vi "ZCAN_InitCAN(PCIeFD ).vi"(4 "error in (no error)":errorcluster caption="错误输入（无错误）", 5 "PCIECANFD系列初始化参数":T1, 6 "can_index":u32, 7 "device_hande":u32) -> (0 "error out":errorcluster caption="错误输出", 2 "can_index_handle":u32)   [LabVIEW 2018]
doc: "用于设置CAN通道的初始化参数。\n\n参数包括：波特率（自定义波特率）、滤波、工作模式；\n\n适用的设备：PCIE-CANFD-100U、PCIE-CANFD-200U、PCIE-CANFD-400U。"
uses:
  zlgcan_labview_20220510/zlgcan_demo_EU/bin/zlgcan_wrap.dll
  data_type/ZCAN_InitCAN_setting_PCIEFD.ctl
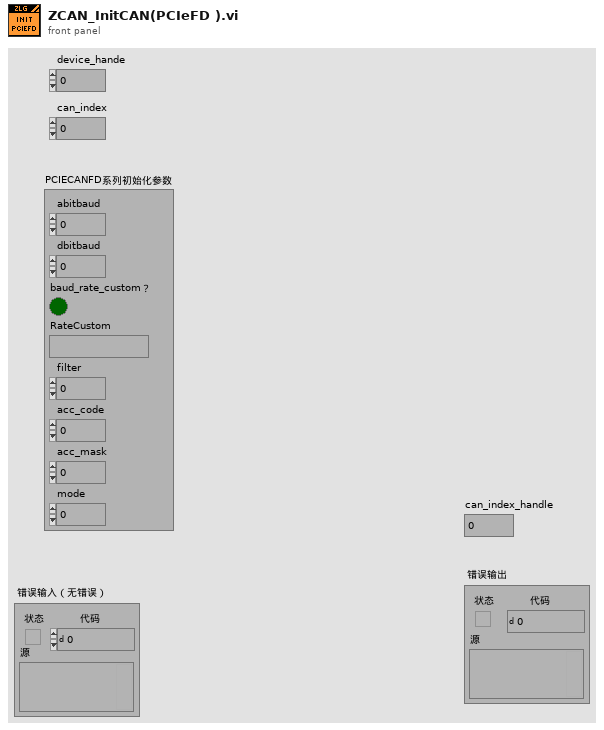
[diagram p1: front panel]
types:
  T1 = typedef "ZCAN_InitCAN_setting_PCIEFD.ctl" = cluster{"abitbaud":u32, "dbitbaud":u32, "baud_rate_custom？":bool, "RateCustom":string, "filter":u8, "acc_code":u32, "acc_mask":u32, "mode":u8}
  T2 = cluster{"can_type":u32, "acc_code":u32, "acc_mask":u32, "can_type":u32, "can_type":u32, "can_type":u32, "filter":u8, u8, "pad":u16, "reserved":u32}
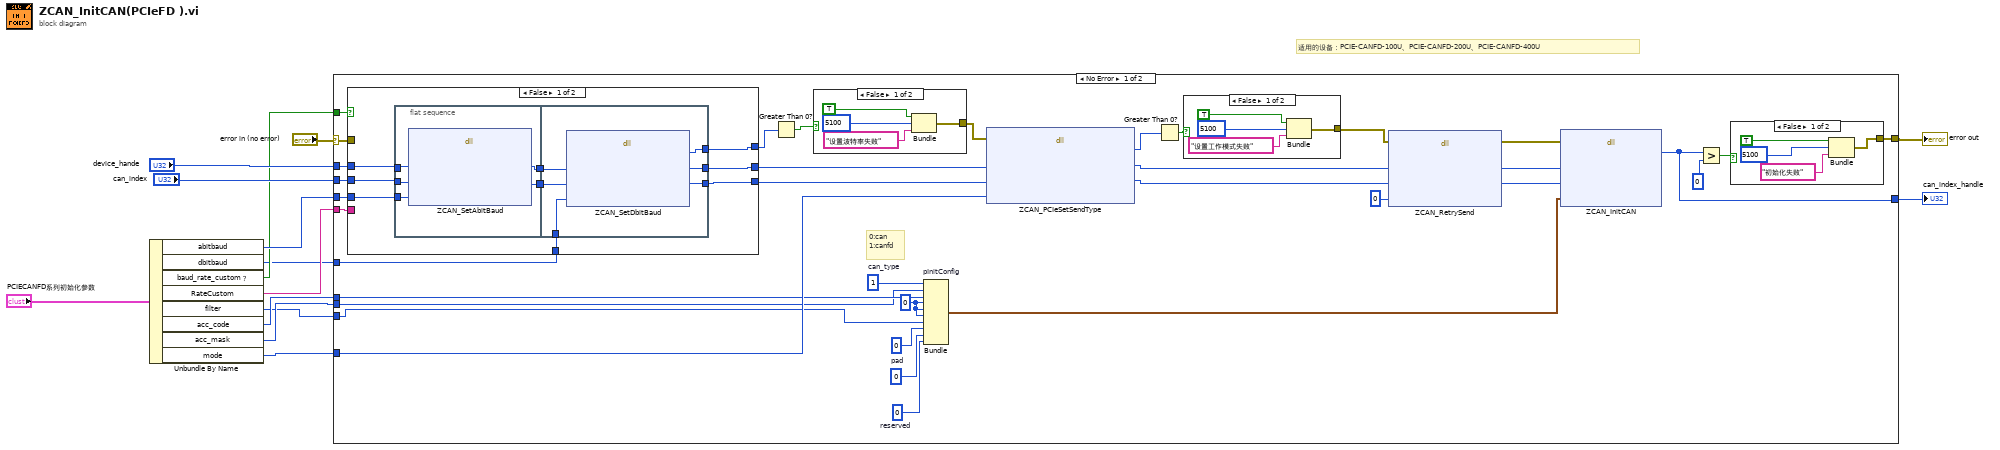
[diagram p0: block diagram]
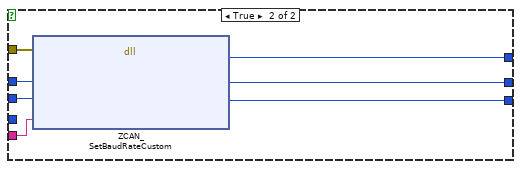
[diagram p5: hidden frame]
diagram:
  # "适用的设备：PCIE-CANFD-100U、PCIE-CANFD-200U、PCIE-CANFD-400U"
  n1 = Unbundle By Name("PCIECANFD系列初始化参数") -> ("abitbaud"=w9:u32, "dbitbaud"=w1:u32, "baud_rate_custom？"=w8:bool, "RateCustom"=w7:string, "filter"=w4:u8, "acc_code"=w6:u32, "acc_mask"=w5:u32, "mode"=w3:u8)
  n2 = case shown="No Error" "error in (no error)" {
    selector: "error in (no error)" -> [w44 w89]
    tunnel: [w40 w89] -> w13
    tunnel: w8 -> [w49 _]
    tunnel: "device_hande" -> [w48 _]
    tunnel: "can_index" -> [w47 _]
    tunnel: w9 -> [w46 _]
    tunnel: w7 -> [w45 _]
    tunnel: [w41 _] -> w12
    tunnel: w6 -> [w18 _]
    tunnel: w5 -> [w17 _]
    tunnel: w4 -> [w16 _]
    tunnel: w3 -> [w39 _]
    tunnel: w1 -> [w15 _]
    frame No Error {
      w22 = u32 0  # reserved
      w23 = u16 0  # pad
      w21 = u32 0 ("can_type")
      w24 = u32 1  # can_type
      # "0:can \n1:canfd"
      n3 = case shown="False" w49 {
        tunnel: w48 -> [w68 w88]
        tunnel: w47 -> [w67 w87]
        tunnel: w46 -> [w66 _]
        tunnel: w45 -> [_ w82]
        tunnel: [w63 w86] -> w37
        tunnel: [w62 w85] -> w38
        tunnel: w44 -> [_ w84]
        tunnel: [w64 w83] -> w36
        tunnel: w15 -> [w65 _]
        frame False {
          n4 = flat-sequence {
            tunnel: w68 -> [w73]
            tunnel: w67 -> [w72]
            tunnel: [w75] -> w70
            tunnel: [w74] -> w69
            tunnel: w66 -> [w71]
            tunnel: w70 -> [w81]
            tunnel: w69 -> [w80]
            tunnel: [w79] -> w64
            tunnel: [w78] -> w63
            tunnel: [w77] -> w62
            tunnel: w65 -> [w76]
            frame #0 {
              n5 = dll-call lib="C:/Users/admin/Desktop/zlgcan_labview_20220510/zlgcan_demo_EU/bin/zlgcan_wrap.dll" fn="ZCAN_SetAbitBaud" label="设置仲裁域波特率"("device_hande"=w73, "can_index"=w72, "abitbaud"=w71) -> ("device_hande"=w75:u32, "can_index"=w74:u32)  [unwired: 5 in, 2 out]
            }
            frame #1 {
              n6 = dll-call lib="C:/Users/admin/Desktop/zlgcan_labview_20220510/zlgcan_demo_EU/bin/zlgcan_wrap.dll" fn="ZCAN_SetDbitBaud" label="设置数据域波特率"("device_hande"=w81, "can_index"=w80, "dbitbaud"=w76) -> ("return"=w79:u32, "device_hande"=w78:u32, "can_index"=w77:u32)  [unwired: 4 in, 2 out]
            }
          }
        }
        frame True {
          n7 = dll-call lib="C:/Users/admin/Desktop/zlgcan_labview_20220510/zlgcan_demo_EU/bin/zlgcan_wrap.dll" fn="ZCAN_SetBaudRateCustom"(error in=w84, "device_handle"=w88, "can_index"=w87, "RateCustom"=w82) -> ("return"=w83:u32, "device_handle"=w86:u32, "can_index"=w85:u32)  [unwired: 3 in, 2 out]
        }
      }
      n8 = Greater Than 0?(x=w36) -> (x > 0?=w35:bool)
      n9 = case shown="False" w35 {
        tunnel: [w58 _] -> w34
        frame False {
          n10 = Bundle("status"=TRUE, "code"=5100, "消息"="设置波特率失败") -> (w58:cluster{"status":bool, "code":i32, "消息":string})  [unwired: 1 in]
        }
        frame True {
        }
      }
      n11 = Bundle "pInitConfig"("can_type"=w24, "acc_code"=w18, "acc_mask"=w17, "can_type"=w21, "can_type"=w21, "can_type"=w21, "filter"=w16, u8 0, "pad"=w23, "reserved"=w22) -> (w19:T2)  [unwired: 1 in]
      n12 = dll-call lib="C:/Users/admin/Desktop/zlgcan_labview_20220510/zlgcan_demo_EU/bin/zlgcan_wrap.dll" fn="ZCAN_PCIeSetSendType" ("ZCAN_SetBaudRateCustom")(error in=w34, "device_handle"=w37, "can_index"=w38, "mode"=w39) -> ("return"=w33:u32, "device_handle"=w28:u32, "can_index"=w27:u32)  [unwired: 3 in, 2 out]
      n13 = Greater Than 0?(x=w33) -> (x > 0?=w32:bool)
      n14 = case shown="False" w32 {
        tunnel: [w50 _] -> w31
        frame False {
          n15 = Bundle("status"=TRUE, "code"=5100, "消息"="设置工作模式失败") -> (w50:cluster{"status":bool, "code":i32, "消息":string})  [unwired: 1 in]
        }
        frame True {
        }
      }
      n16 = dll-call lib="C:/Users/admin/Desktop/zlgcan_labview_20220510/zlgcan_demo_EU/bin/zlgcan_wrap.dll" fn="ZCAN_RetrySend" ("ZCAN_SetBaudRateCustom")(error in=w31, "device_handle"=w28, "can_index"=w27, "retry_send"=u32 0) -> (error out=w29:errorcluster, "device_handle"=w26:u32, "can_index"=w25:u32)  [unwired: 4 in, 1 out]
      n17 = dll-call lib="C:/Users/admin/Desktop/zlgcan_labview_20220510/zlgcan_demo_EU/bin/zlgcan_wrap.dll" fn="ZCAN_InitCAN"(error in=w29, "device_handle"=w26, "can_index"=w25, "pInitConfig"=w19) -> ("can_handle"=w41:u32)  [unwired: 5 in, 2 out]
      n18 = Greater?(x=w41, y=0) -> (0:w42:bool)
      n19 = case shown="False" w42 {
        tunnel: [w54 _] -> w40
        frame False {
          n20 = Bundle("status"=TRUE, "code"=5100, "消息"="初始化失败") -> (w54:cluster{"status":bool, "code":i32, "消息":string})  [unwired: 1 in]
        }
        frame True {
        }
      }
    }
    frame Error {
    }
  }
  "error out" <- w13
  "can_index_handle" <- w12
